vi "Make_Array_of_Tracks-1.vi"(4 "error IN":errorcluster, 6 "[IN] Filtered Tracks w/t Problems":T1(array[cluster]), 7 "[IN] Filtered Tracks with Problems":T1(array[cluster])) -> (0 "error OUT":errorcluster, 2 "[OUT] Array of tracks":cluster{"Tracks":dbl[], "Start Pos":i32}[](array[cluster]))   [LabVIEW 2017]
doc: "Merging 2 arrays of clusters with tracks into 1 array of cluster (e.g. for further path velocity calculation)"
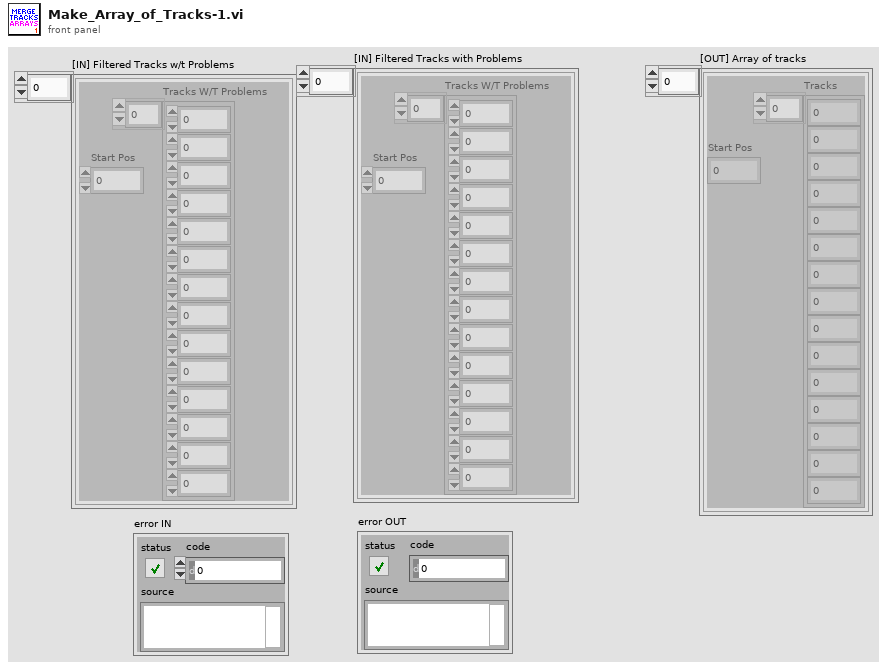
[diagram p1: front panel]
types:
  T1 = cluster{"Tracks W/T Problems":dbl[], "Start Pos":i32}[]
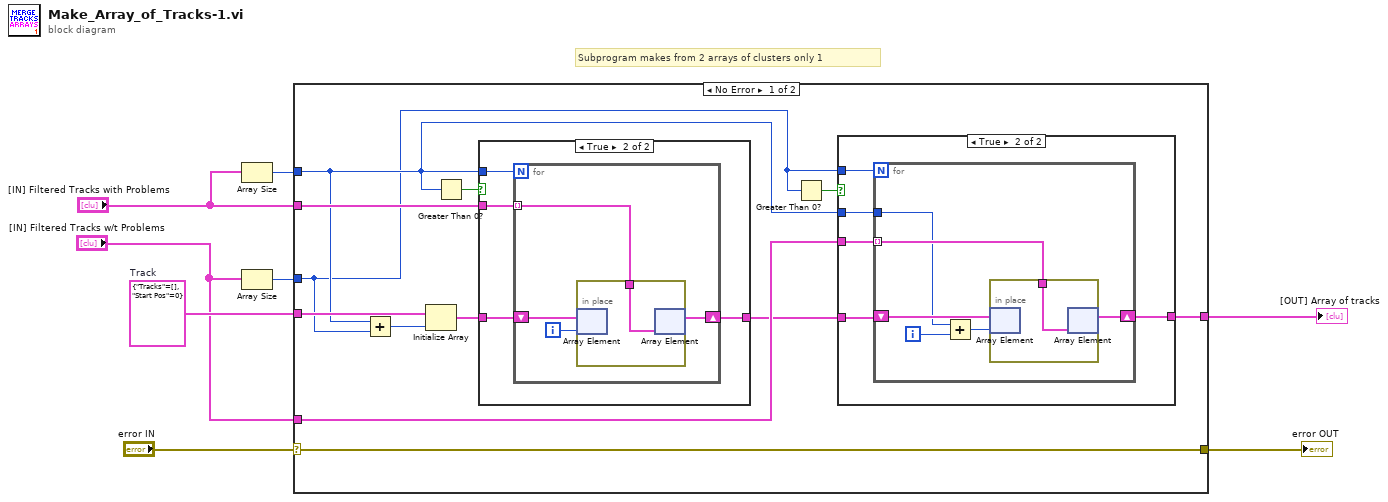
[diagram p0: block diagram]
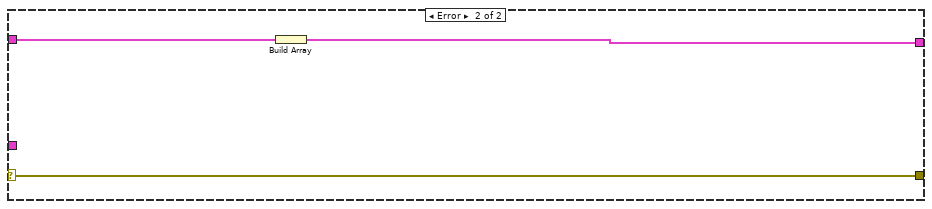
[diagram p4: hidden frame]
diagram:
  w8 = cluster{"Tracks":dbl[], "Start Pos":i32} {"Tracks"=[], "Start Pos"=0}  # Track
  # "Subprogram makes from 2 arrays of clusters only 1"
  n1 = Array Size(array="[IN] Filtered Tracks with Problems") -> (size(s)=w4:i32)
  n2 = Array Size(array="[IN] Filtered Tracks w/t Problems") -> (size(s)=w5:i32)
  n3 = case shown="No Error" "error IN" {
    selector: "error IN" -> [w12 w44]
    tunnel: w8 -> [w20 w46]
    tunnel: "[IN] Filtered Tracks with Problems" -> [w17 _]
    tunnel: "[IN] Filtered Tracks w/t Problems" -> [w16 _]
    tunnel: w5 -> [w10 _]
    tunnel: w4 -> [w13 _]
    tunnel: [w12 w44] -> w2
    tunnel: [w14 w45] -> w1
    frame No Error {
      n4 = Add(x=w13, y=w10) -> (x+y=w19:i32)
      n5 = Initialize Array(w20, w19) -> (w18:cluster{"Tracks":dbl[], "Start Pos":i32}[])
      n6 = Greater Than 0?(x=w13) -> (x > 0?=w11:bool)
      n7 = case shown="True" w11 {
        tunnel: w18 -> [w34 w38]
        tunnel: w17 -> [_ w37]
        tunnel: [w34 w36] -> w15
        tunnel: w13 -> [_ w35]
        frame False {
        }
        frame True {
          n8 = for {
            N: w35 -> [_]
            shift-right: [w39] -> w36
            shift-left: w38 -> [w42]
            tunnel: w37 -> [w40] mode=indexing
            i -> [w41]
            n9 = in-place {
              in-place-border: w40 -> [w43]
              n10 = in-place-array #1(w42, w41) -> ()  [unwired: 1 out]
              n11 = in-place-array #1(w43) -> (w39:cluster{"Tracks":dbl[], "Start Pos":i32}[])  [unwired: 1 out]
            }
          }
        }
      }
      n12 = Greater Than 0?(x=w10) -> (x > 0?=w9:bool)
      n13 = case shown="True" w9 {
        tunnel: w16 -> [_ w26]
        tunnel: w15 -> [w21 w25]
        tunnel: w10 -> [_ w24]
        tunnel: [w21 w23] -> w14
        tunnel: w13 -> [_ w22]
        frame False {
        }
        frame True {
          n14 = for {
            N: w24 -> [_]
            shift-right: [w30] -> w23
            shift-left: w25 -> [w32]
            tunnel: w26 -> [w31] mode=indexing
            tunnel: w22 -> [w27]
            i -> [w29]
            n15 = Add(x=w27, y=w29) -> (x+y=w28:i32)
            n16 = in-place {
              in-place-border: w31 -> [w33]
              n17 = in-place-array #2(w32, w28) -> ()  [unwired: 1 out]
              n18 = in-place-array #2(w33) -> (w30:cluster{"Tracks":dbl[], "Start Pos":i32}[])  [unwired: 1 out]
            }
          }
        }
      }
    }
    frame Error {
      n19 = Build Array(w46) -> (w45:cluster{"Tracks":dbl[], "Start Pos":i32}[])
    }
  }
  "error OUT" <- w2
  "[OUT] Array of tracks" <- w1
